vi "Do.vi"(8 "error in (no error)":errorcluster, 10 "Actor in":refnum<class "Actor.lvclass">, 11 "Conceret Set Create Test Node Key Focus Msg in":refnum<class "Conceret Set Create Test Node Key Focus Msg.lvclass">) -> (0 "error out":errorcluster, 2 "Actor out":refnum<class "Actor.lvclass">)   [LabVIEW 2013, in "Create Test Node View.lvlib" / "Conceret Set Create Test Node Key Focus Msg.lvclass"]
doc: "(<B>Filename</B>: Actor Framework.lvlib:Message.lvclass:Do.vi)\n\nDefines what a message does when it is received by an actor. Generally, a message instructs an actor to invoke one of its methods.\n\nBy default, this method does nothing. A child class must override it to define behavior. Create a child class by using the Actor Framework Message Maker dialog box."
uses:
  Conceret Set Create Test Node Key Focus Msg.lvclass
  <vilib>/ActorFramework/Actor/Actor.lvclass
  Create Test Node View/Create Test Node View.lvclass
  Models/Create Test Node Model Messages/Abstract Set Create Test Node Key Focus Msg/Abstract Set Create Test Node Key Focus Msg.lvclass
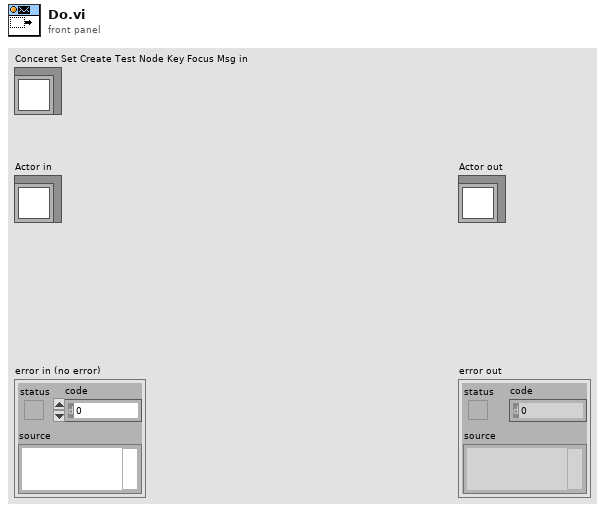
[diagram p1: front panel]
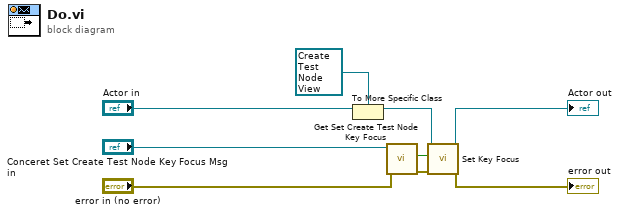
[diagram p0: block diagram]
diagram:
  n1 = To More Specific Class(target class=refnum<class "Create Test Node View.lvclass"> refnum ("Create Test Node View.lvlib:Create Test Node View.lvclass"), reference="Actor in") -> (specific class reference=w6:refnum<class "Create Test Node View.lvclass">)  [unwired: 1 in, 1 out]
  n2 = call "Get Set Create Test Node Key Focus.vi"("error in (no error)"="error in (no error)", "Abstract Set Create Test Node Key Focus Msg in"="Conceret Set Create Test Node Key Focus Msg in") -> ("error out"=w5:errorcluster, "Set Create Test Node Key Focus"=w1:bool)  [unwired: 7 in, 1 out]
  n3 = call "Set Key Focus.vi"("error in (no error)"=w5, "Set Create Test Node Key Focus"=w1, "Create Test Node View in"=w6) -> ("error out"=→"error out":errorcluster, "Create Test Node View out"=→"Actor out":refnum<class "Create Test Node View.lvclass">)  [unwired: 7 in]
